vi "RubikTurn.vi"(3 "error in":errorcluster, 4 "Turn":T1=enum."ccw", 5 "Servo":T2) -> (0 "error out":errorcluster, 1 "Servo Angle\n Status":enum16{"+90°", "0°", "-90°"}(ring)=enum."-90°")   [LabVIEW 2017]
uses:
  Projekt-RubikLibrary/ServoEnumControl.ctl
  Projekt-RubikLibrary/ServoCCWControl.ctl
  Projekt-RubikLibrary/RubikLibrary.lvlib
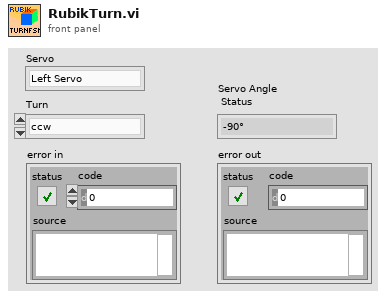
[diagram p1: front panel]
types:
  T1 = typedef "RubikLibrary.lvlib/ServoCCWControl.ctl" = enum16{"cw", "ccw"}
  T2 = typedef "RubikLibrary.lvlib/ServoEnumControl.ctl" = enum16{"Left Servo", "Front Servo", "Right Servo"}
  T3 = typedef "RubikLibrary.lvlib/ServoAbsAngleControl.ctl" = enum16{"+90°", "0°", "-90°"}
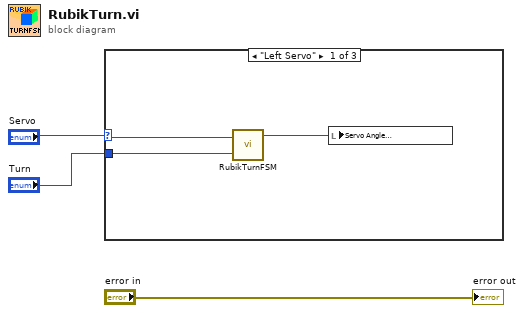
[diagram p0: block diagram]
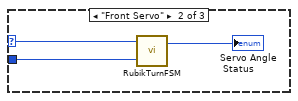
[diagram p2: hidden frame]
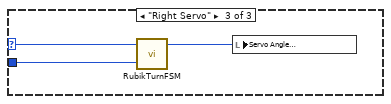
[diagram p3: hidden frame]
diagram:
  n1 = case shown="\"Left Servo\"" "Servo" {
    selector: "Servo" -> [w6 w7 w12]
    tunnel: "Turn" -> [w5 w9 w11]
    frame "Left Servo" {
      n2 = call "RubikTurnFSM.vi"("Turn"=w5, "Servo Enum"=w6) -> ("Turn State (out)"=w4:T3)
      n3 = local write "Servo Angle\n Status"(w4) -> ()
    }
    frame "Front Servo" {
      n4 = call "RubikTurnFSM.vi"("Turn"=w9, "Servo Enum"=w7) -> ("Turn State (out)"=→"Servo Angle\n Status":T3)
    }
    frame "Right Servo" {
      n5 = call "RubikTurnFSM.vi"("Turn"=w11, "Servo Enum"=w12) -> ("Turn State (out)"=w10:T3)
      n6 = local write "Servo Angle\n Status"(w10) -> ()
    }
  }
  "error out" <- "error in"
